vi "Com Config Serial.vi"(8 "error in (no error)":errorcluster, 11 "VISA Refnum in":refnum<visa-resource-name>) -> (0 "error out":errorcluster, 3 "VISA Refnum out":refnum<visa-resource-name>)   [LabVIEW 2016, in "SR7270 Drivers.lvlib"]
uses:
  SR7270 Drivers.lvlib
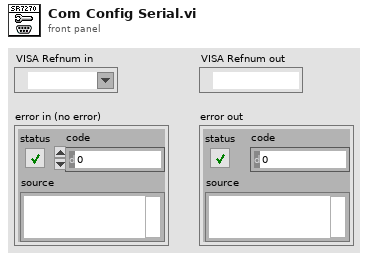
[diagram p1: front panel]
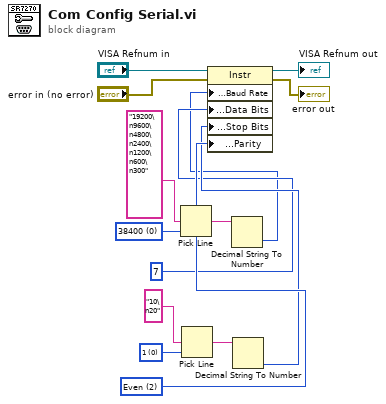
[diagram p0: block diagram]
diagram:
  w14 = u8 2 items=["None", "Odd", "Even"] ("Parity")
  w9 = u8 0 items=["1", "2"] ("Stop Bits")
  w6 = u16 0 items=["38400", "19200", "9600", "4800", "2400", "1200", "600", "300"] ("Baud Rate")
  n1 = Pick Line(multi-line string="19200\n9600\n4800\n2400\n1200\n600\n300", line index=w6) -> (output string=w10:string)  [unwired: 1 in]
  n2 = Pick Line(multi-line string="10\n20", line index=w9) -> (output string=w8:string)  [unwired: 1 in]
  n3 = Decimal String To Number(string=w10) -> (number=w11:i32)  [unwired: 2 in, 1 out]
  n4 = Decimal String To Number(string=w8) -> (number=w13:i32)  [unwired: 2 in, 1 out]
  n5 = property class="Instr"(reference="VISA Refnum in", error in="error in (no error)", "Serial Settings:Baud Rate"=w11, "Serial Settings:Data Bits"=u8 7 ("Data Bits"), "Serial Settings:Stop Bits"=w13, "Serial Settings:Parity"=w14) -> (reference out=→"VISA Refnum out":refnum<visa-resource-name>, error out=→"error out":errorcluster)
